vi "ReadIncrementSerialRegistryKey.vi"() -> (3 "CurrentID":i32)   [LabVIEW 2017]
uses:
  <vilib>/registry/registry.llb/Registry RtKey.ctl
  <vilib>/registry/registry.llb/Read Registry Value Simple STR.vi
  <vilib>/registry/registry.llb/Write Registry Value Simple STR.vi
panel:
  out "Date Checker":bool
  out "Last used Serial  2":string
  out "error out":errorcluster
  out "Last used Serial":string
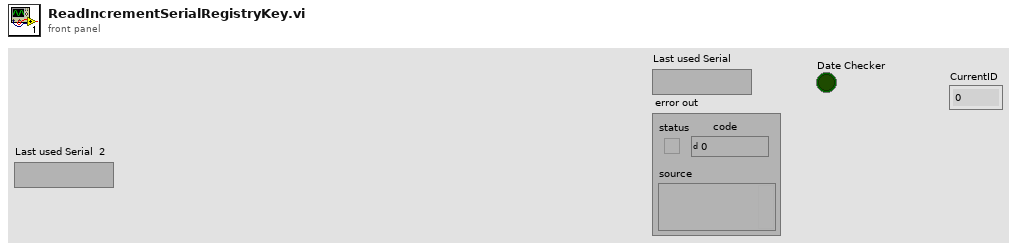
[diagram p1: front panel]
types:
  T1 = typedef "Registry RtKey.ctl" = enum32{"HKEY_CLASSES_ROOT", "HKEY_CURRENT_USER", "HKEY_LOCAL_MACHINE", "HKEY_USERS", "HKEY_PERFORMANCE_DATA", "HKEY_CURRENT_CONFIG", "HKEY_DYN_DATA"}
  T2 = typedef "Registry refnum.ctl" = refnum<k1>
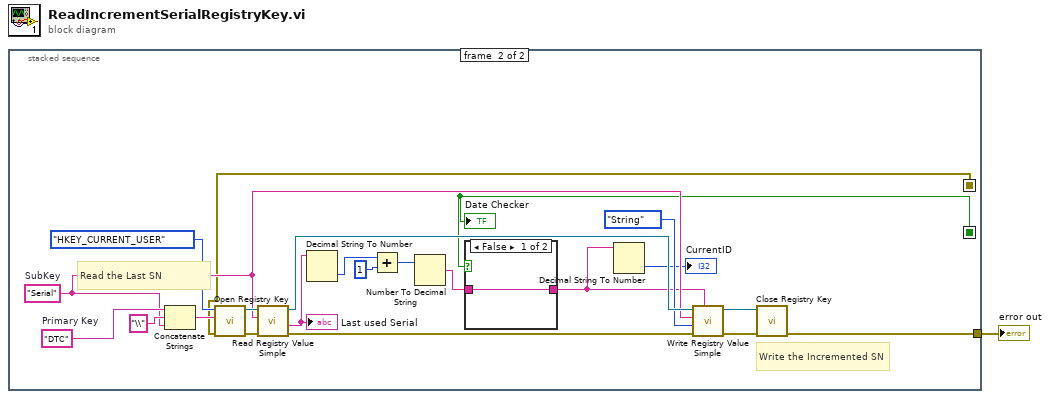
[diagram p0: block diagram]
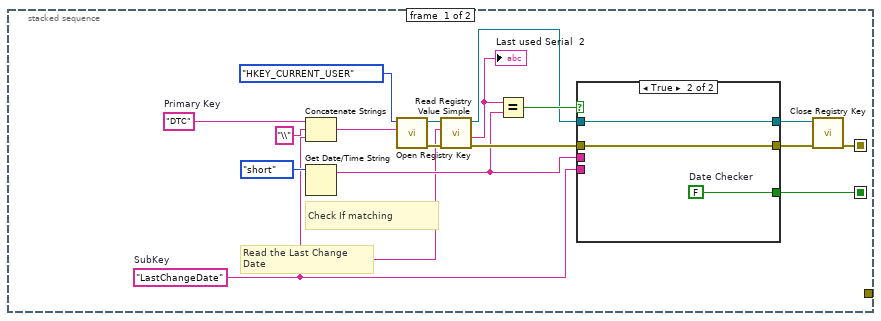
[diagram p2: hidden frame]
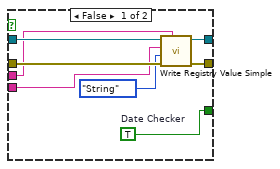
[diagram p3: hidden frame]
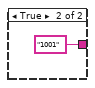
[diagram p4: hidden frame]
diagram:
  n1 = stacked-sequence {
    seq-local: [w3 _] -> [_ w34]
    seq-local: [w2 _] -> [_ w32]
    tunnel: [_ w33] -> w1
    frame #0 {
      w4 = "LastChangeDate"  # SubKey
      w15 = "DTC"  # Primary Key
      # "Check If matching"
      # "Read the Last Change Date"
      n2 = Concatenate Strings(w15, "\\" ("string"), w4) -> (w13:string)
      n3 = Get Date/Time String(date format (0)=enum16{"short", "long", "abbreviated"}."short") -> (date string=w5:string)  [unwired: 2 in, 1 out]
      n4 = call <vilib>:"Open Registry Key.vi"("subkey"=w13, "root key (HKEY_LOCAL_MACHINE)"=Registry_RtKey."HKEY_CURRENT_USER") -> ("error out"=w17:errorcluster, "refnum out"=w18:T2)  [unwired: 8 in]
      n5 = call-poly <vilib>:"Read Registry Value Simple.vi"("error in (no error)"=w17, "value"=w4, "refnum"=w18) -> ("error out"=w9:errorcluster, "String/Binary data"=w11:string, "refnum out"=w8:T2)  [unwired: 3 in, 1 out]
      "Last used Serial  2" <- w11
      n6 = Equal?(x=w11, y=w5) -> (x = y?=w10:bool)
      n7 = case shown="True" w10 {
        tunnel: w9 -> [w25 w28]
        tunnel: w8 -> [w26 w29]
        tunnel: [w21 w29] -> w7
        tunnel: [w22 w28] -> w6
        tunnel: w5 -> [w24 _]
        tunnel: w4 -> [w23 _]
        tunnel: [w20 w27] -> w2
        frame False {
          w20 = TRUE  # Date Checker
          n8 = call-poly <vilib>:"Write Registry Value Simple.vi"("String/Binary data"=w24, "error in (no error)"=w25, "simple data type"=enum16{"String", "Binary", "DWORD"}."String", "value"=w23, "refnum"=w26) -> ("error out"=w22:errorcluster, "refnum out"=w21:T2)  [unwired: 3 in]
        }
        frame True {
          w27 = FALSE  # Date Checker
        }
      }
      n9 = call <vilib>:"Close Registry Key.vi"("error in (no error)"=w6, "refnum"=w7) -> ("error out"=w3:errorcluster)  [unwired: 5 in]
    }
    frame #1 {
      w37 = "Serial"  # SubKey
      w48 = "DTC"  # Primary Key
      # "Write the Incremented SN"
      # "Read the Last SN"
      n10 = Concatenate Strings(w48, "\\" ("string"), w37) -> (w46:string)
      n11 = call <vilib>:"Open Registry Key.vi"("error in (no error)"=w34, "subkey"=w46, "root key (HKEY_LOCAL_MACHINE)"=Registry_RtKey."HKEY_CURRENT_USER") -> ("error out"=w50:errorcluster, "refnum out"=w51:T2)  [unwired: 7 in]
      n12 = call-poly <vilib>:"Read Registry Value Simple.vi"("error in (no error)"=w50, "value"=w37, "refnum"=w51) -> ("error out"=w45:errorcluster, "String/Binary data"=w41:string, "refnum out"=w42:T2)  [unwired: 3 in, 1 out]
      "Last used Serial" <- w41
      n13 = Decimal String To Number(string=w41) -> (number=w40:i32)  [unwired: 2 in, 1 out]
      n14 = Add(x=w40, y=1) -> (x+y=w38:i32)
      n15 = Number To Decimal String(number=w38) -> (decimal integer string=w31:string)  [unwired: 1 in]
      n16 = case shown="False" w32 {
        tunnel: [w52 "1001"] -> w30
        tunnel: w31 -> [w52 _]
        frame False {
        }
        frame True {
        }
      }
      n17 = Decimal String To Number(string=w30) -> (number=→"CurrentID":i32)  [unwired: 2 in, 1 out]
      n18 = call-poly <vilib>:"Write Registry Value Simple.vi"("String/Binary data"=w30, "error in (no error)"=w45, "simple data type"=enum16{"String", "Binary", "DWORD"}."String", "value"=w37, "refnum"=w42) -> ("error out"=w44:errorcluster, "refnum out"=w43:T2)  [unwired: 3 in]
      n19 = call <vilib>:"Close Registry Key.vi"("error in (no error)"=w44, "refnum"=w43) -> ("error out"=w33:errorcluster)  [unwired: 5 in]
      "Date Checker" <- w32
    }
  }
  "error out" <- w1
